vi "Write J_count.vi"(8 "error in (no error)":errorcluster, 10 "J/count":dbl[unit], 11 "Analyze Parameter Energy per Count in":refnum<class "Analyze Parameter Energy per Count.lvclass">) -> (0 "error out":errorcluster, 3 "Analyze Parameter Energy per Count out":refnum<class "Analyze Parameter Energy per Count.lvclass">)   [LabVIEW 2014, in "Analyze Parameter Energy per Count.lvclass"]
uses:
  Analyze Parameter Energy per Count.lvclass
  Analyze Parameter Energy per Count.lvclass/Analyze Parameter Energy per Count.ctl
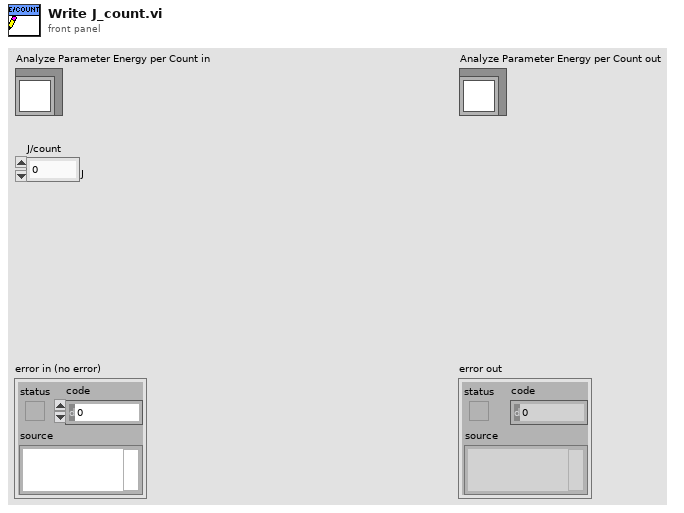
[diagram p1: front panel]
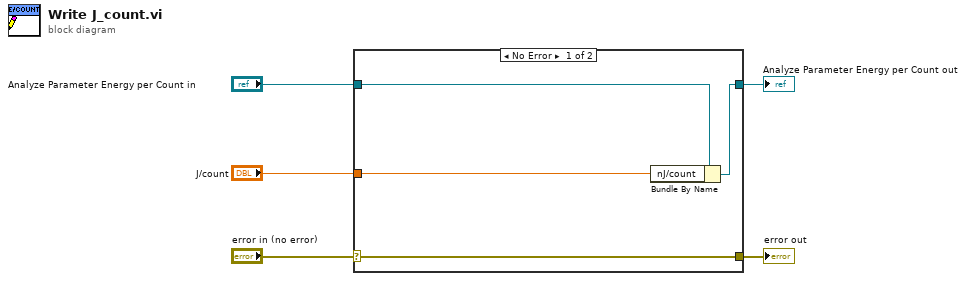
[diagram p0: block diagram]
diagram:
  n1 = case shown="No Error" "error in (no error)" {
    selector: "error in (no error)" -> [w9 w10]
    tunnel: [w9 w10] -> w4
    tunnel: [w7 w11] -> w2
    tunnel: "Analyze Parameter Energy per Count in" -> [w8 w11]
    tunnel: "J/count" -> [w6 _]
    frame No Error {
      n2 = Bundle By Name(cluster=w8, "nJ/count"=w6) -> (w7:refnum<class "Analyze Parameter Energy per Count.lvclass">)
    }
    frame Error {
    }
  }
  "error out" <- w4
  "Analyze Parameter Energy per Count out" <- w2
